vi "Begin.vi"(11 "Image Size":T1=enum."320x240") -> (0 "error out":errorcluster)   [LabVIEW 2012]
doc: "Called before other user functions, this VI is expected to open initial I/O refnums, load in file data, and do all program initialization. Notice that the <B>error out</B> terminal is simply used for data flow. Wiring it to other structures or subVIs ensures that this VI runs first."
uses:
  <vilib>/Rock Robotics/WPI/Camera/WPI_CameraImageSize.ctl
  <vilib>/Rock Robotics/WPI/DriverStation/WPI_DriverStationRobotMode2.ctl
  <vilib>/Rock Robotics/WPI/Joystick/WPI_JoystickDeviceEnum.ctl
  <vilib>/Rock Robotics/SystemInterfaces/DIO/FPGA_DIOPWMChannel.ctl
  <vilib>/Rock Robotics/SystemInterfaces/DIO/FPGA_DIORelayChannel.ctl
  <vilib>/Rock Robotics/SystemInterfaces/DIO/FPGA_DIOChannel.ctl
  <vilib>/Rock Robotics/SystemInterfaces/Typedef/FPGA_TypedefDigitalModule.ctl
  <vilib>/Rock Robotics/WPI/Encoder/WPI_EncoderType.ctl
  <vilib>/Rock Robotics/WPI/Solenoid/WPI_SolenoidChannel.ctl
  <vilib>/Rock Robotics/SystemInterfaces/Typedef/FPGA_TypedefAnalogModule.ctl
  <vilib>/Rock Robotics/SystemInterfaces/AI/FPGA_AIChannel.ctl
  RefnameEnum.ctl
  Sally_Dashboard_2014/DBNameEnum.ctl
  <vilib>/Rock Robotics/WPI/Solenoid/WPI_SolenoidValue.ctl
  <vilib>/Rock Robotics/WPI/SafetyOutput/WPI_SafetyOutputConfigMenu.ctl
  <vilib>/Rock Robotics/SystemInterfaces/CounterEncoderSourceConvertion/FPGA_CounterEncoderSourceConvertionLVSourceType.ctl
  <vilib>/Rock Robotics/SystemInterfaces/DIO/FPGA_DIODigitalSourceChannel.ctl
  <vilib>/Rock Robotics/SystemInterfaces/AnalogTrigger/FPGA_AnalogTriggerIndex.ctl
  <vilib>/Rock Robotics/SystemInterfaces/AnalogTrigger/FPGA_AnalogTriggerOutType.ctl
  Robot Global Data.vi
  <vilib>/Rock Robotics/WPI/RobotDrive/WPI_RobotDriveOpen2MotorWithTalon.vi
  <vilib>/Rock Robotics/WPI/MotorControl/WPI_MotorControlOpen Talon.vi
  <vilib>/Rock Robotics/WPI/Counter/WPI_CounterDigitalInputToDigitalSource.vi
  <vilib>/Rock Robotics/WPI/Solenoid/WPI_SolenoidOpenSingle.vi
  <vilib>/Rock Robotics/WPI/Solenoid/WPI_SolenoidSetEnum.vi
  <vilib>/Rock Robotics/WPI/MotorControl/WPI_MotorControlOpen Jaguar.vi
  <vilib>/Rock Robotics/WPI/Compressor/WPI_CompressorGetSetRefNum.vi
  <vilib>/Rock Robotics/WPI/Counter/WPI_CounterOpen UpDown Mode.vi
  <vilib>/Rock Robotics/WPI/Camera/WPI_CameraWhite Balance Values.ctl
  <vilib>/Rock Robotics/WPI/Camera/WPI_CameraExposure Values.ctl
  <vilib>/Rock Robotics/WPI/Camera/WPI_CameraFrameRate.ctl
  <vilib>/Rock Robotics/SystemInterfaces/Typedef/FPGA_TypedefAnalogModuleForGyro.ctl
  <vilib>/Rock Robotics/SystemInterfaces/AI/FPGA_AIGyroChannel.ctl
panel:
  in  "LowerLimit (v)":dbl=-1.0
  in  "UpperLimit (v)":dbl=1.0
  out "error out 2":errorcluster
  in  "Version String":string="TruongFramework 1.42"
  # "DON'T FORGET TO MAKE THIS DEFAULT"
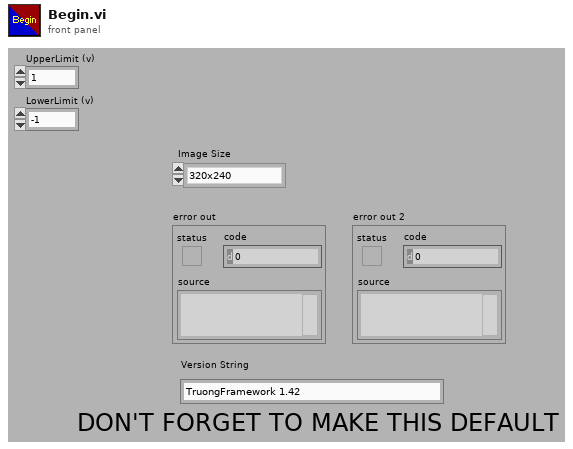
[diagram p1: front panel]
types:
  T1 = typedef "WPI_CameraImageSize.ctl" = enum16{"640x480", "320x240", "160x120"}
  T2 = typedef "WPI_SafetyOutputConfigMenu.ctl" = enum16{"Enable", "Disable"}
  T3 = typedef "WPI_SolenoidValue.ctl" = enum16{"Off", "On", "Forward", "Reverse"}
  T4 = typedef "RefnameEnum.ctl" = enum16{"FireLauncher", "Climber", "Shield", "TankDrive", "DriveEncoderL", "DriveEncoderR", "LauncherMotorRPM", "LauncherEncoderAnalog", "LauncherEncoderRPM", "ShooterLS", "DriveAlignLSLeft", "DriveAlignLSRight", "ClimbingLS", "LauncherEncoderAngle", "LauncherMotorAngle", "Gamepad1", "Gamepad2", "Compressor", "ClimbWeightSol3", "ClimbWeightSol4"}
  T5 = typedef "WPI_SolenoidChannel.ctl" = enum8{"Solenoid 1", "Solenoid 2", "Solenoid 3", "Solenoid 4", "Solenoid 5", "Solenoid 6", "Solenoid 7", "Solenoid 8", "Invalid"}
  T6 = typedef "FPGA_DIOChannel.ctl" = enum8{"DIO 1", "DIO 2", "DIO 3", "DIO 4", "DIO 5", "DIO 6", "DIO 7", "DIO 8", "DIO 9", "DIO 10", "DIO 11", "DIO 12", "DIO 13", "DIO 14", "Invalid"}
  T7 = typedef "FPGA_TypedefDigitalModule.ctl" = enum16{"Digital Module 1", "Digital Module 2"}
  T8 = typedef "DBNameEnum.ctl" = enum16{"AutoInstructions", "DriveLoopTime", "DriveAlignLSLeft", "DriveAlignLSRight", "Use2DriveAlign", "ClimbLS", "LauncherAngleMatches", "FrameworkVersion", "sLauncherAngle", "LauncherTargetAngle", "sLauncherRPM", "LauncherTargetRPM", "sDriveDistance", "LauncherMotorValue", "PullbackTol", "FireTol", "LauncherRPMTol", "LauncherAngleTol", "InitialWait", "WaitBetweenLaunch", "AnglePresets", "RPMPresets", "UseAngleEncoder", "UseLauncherEncoder", "UseLauncherPID", "QSWaitBeforeFire", "QSWaitBeforeRetract", "AngleForwardValue", "AngleBackwardValue", "UseClusterArray", "BackupAuto", "ReverseDriveIndicate", "HalfSpeedFactor"}
  T9 = typedef "FPGA_AIChannel.ctl" = enum8{"AI 1", "AI 2", "AI 3", "AI 4", "AI 5", "AI 6", "AI 7", "AI 8", "Invalid"}
  T10 = typedef "FPGA_TypedefAnalogModule.ctl" = enum16{"Analog Module 1", "Analog Module 2"}
  T11 = typedef "WPI_EncoderType.ctl" = enum16{"1x", "2x", "4x"}
  T12 = typedef "FPGA_DIORelayChannel.ctl" = enum8{"Relay 1", "Relay 2", "Relay 3", "Relay 4", "Relay 5", "Relay 6", "Relay 7", "Relay 8", "Invalid"}
  T13 = typedef "FPGA_DIOPWMChannel.ctl" = enum8{"PWM 1", "PWM 2", "PWM 3", "PWM 4", "PWM 5", "PWM 6", "PWM 7", "PWM 8", "PWM 9", "PWM 10", "Invalid"}
  T14 = typedef "WPI_JoystickDeviceEnum.ctl" = enum16{"USB 1", "USB 2", "USB 3", "USB 4", "Kinect 1", "Kinect 2"}
  T15 = typedef "WPI_DriverStationRobotMode2.ctl" = enum16{"Autonomous Disabled", "Autonomous Enabled", "Teleop Disabled", "Teleop Enabled", "Timeout", "Finish", "Test Disabled", "Test Enabled"}
  T16 = enum16{"Rising Edge", "Falling Edge", "Raising & Falling Edge", "Disabled"}
  T17 = typedef "WPI_DigitalInputDevRef.ctl" = cluster{"DevStatus":errorcluster, "DIO Channel":T6, "Digital Module":T7}
  T18 = typedef "FPGA_CounterEncoderSourceConvertionLVSourceType.ctl" = cluster{"DevStatus":errorcluster, "AnalogTriggerMode?":bool, "DigitalMode":cluster{"Digital Module":T7, "DIO Channel":T19}, "AnalogTriggerMode":cluster{"AnalogTriggerIndex":T20, "OutputType":T21}}
  T19 = typedef "FPGA_DIODigitalSourceChannel.ctl" = enum8{"DIO 1", "DIO 2", "DIO 3", "DIO 4", "DIO 5", "DIO 6", "DIO 7", "DIO 8", "DIO 9", "DIO 10", "DIO 11", "DIO 12", "DIO 13", "DIO 14", "Disabled"}
  T20 = typedef "FPGA_AnalogTriggerIndex.ctl" = enum8{"Trig 0", "Trig 1", "Trig 2", "Trig 3", "Trig 4", "Trig 5", "Trig 6", "Trig 7", "Invalid"}
  T21 = typedef "FPGA_AnalogTriggerOutType.ctl" = enum16{"InWindow", "TriggerState", "Rising", "Falling"}
  T22 = typedef "WPI_EncoderDevRef.ctl" = cluster{"DevStatus":errorcluster, "EncoderIndex":T23, "CounterIndex":T24, "DistancePerCount":dbl, "Decoding Type":T11}
  T23 = typedef "FPGA_EncoderIdx.ctl" = enum8{"Enc 0", "Enc 1", "Enc 2", "Enc 3", "Invalid"}
  T24 = typedef "FPGA_CounterCtrSystemIndex.ctl" = enum8{"Ctr 0", "Ctr 1", "Ctr 2", "Ctr 3", "Ctr 4", "Ctr 5", "Ctr 6", "Ctr 7", "Invalid"}
  T25 = typedef "WPI_CounterDevRef.ctl" = cluster{"DevStatus":errorcluster, "CntIndex":T24}
  T26 = typedef "FPGA_AIGyroChannel.ctl" = enum8{"AI 1", "AI 2", "Invalid"}
  T27 = typedef "FPGA_TypedefAnalogModuleForGyro.ctl" = enum16{"Analog Module 1"}
  T28 = typedef "WPI_GyroDevRef.ctl" = cluster{"DevStatus":errorcluster, "Analog Module":T10, "Analog Channel":T9, "Offset":dbl, "Gain (VoltsPerDegree/Second)":dbl}
  T29 = typedef "WPI_MotorControlDeviceRef.ctl" = cluster{"DeviceStatus":errorcluster, "Type":enum16{"PWM", "CAN"}, "PWM":cluster{"Digital Module":T7, "PWM Channel":T13, "DeadBand":T30}, "CAN":cluster{"Device Number":u8, "Control Mode":T31, "Semaphore":T32, "Max Vout":dbl}, "Invert":bool, "TransformRef":T33, "InvTransformRef":T33}
  T30 = typedef "WPI_PWMDeadband.ctl" = cluster{"Name":string, "maxPositivePwm":i32, "minPositivePwm":i32, "centerPwm":i32, "maxNegativePwm":i32, "minNegativePwm":i32, "angularRange":u16}
  T31 = typedef "WPI_CANJaguar_ControlMode.ctl" = enum8{"Percent VBus", "Current", "Speed", "Position", "Voltage"}
  T32 = typedef "Semaphore RefNum" = refnum<k1>
  T33 = typedef "WPI_PWMTransform_ConPane.ctl" = refnum<vi>
  T34 = typedef "WPI_RelayDevRef.ctl" = cluster{"DevStatus":errorcluster, "Relay Channel":T12, "Digital Module":T7, "Relay Direction":T35}
  T35 = typedef "WPI_RelayDirection.ctl" = enum16{"Both directions", "Forward only", "Reverse only"}
  T36 = typedef "WPI_SolenoidDevRef.ctl" = cluster{"DevStatus":errorcluster, "Solenoid Module":T37, "Forward Solenoid Channel":T5, "Reverse Solenoid Channel":T5}
  T37 = typedef "FPGA_TypedefSolenoidModule.ctl" = enum16{"Solenoid Module 1", "Solenoid Module 2"}
  T38 = typedef "WPI_CompressorDevRef.ctl" = cluster{"DevStatus":errorcluster, "DigitalInputDevRef":T17, "RelayDevRef":T34}
  T39 = typedef "WPI_RobotDriveDevRef.ctl" = cluster{"DevStatus":errorcluster, "Motors[]":T29[], "Square Inputs":bool, "Max Output":dbl, "Isochronous":bool}
  T40 = typedef "WPI_CameraFrameRate.ctl" = u32
  T41 = typedef "WPI_CameraExposure Values.ctl" = enum16{"Auto", "Flicker-free 50 Hz", "Flicker-free 60 Hz", "Hold current"}
  T42 = typedef "WPI_CameraWhite Balance Values.ctl" = enum16{"Auto", "Fixed indoor", "Fixed outdoor 1", "Fixed outdoor 2", "Fixed fluorescent 1", "Fixed fluorescent 2", "Hold current"}
  T43 = typedef "WPI_CameraDevRef.ctl" = cluster{"Camera Address":string, "CameraStatus":errorcluster, "Acquire Image Notifier":refnum<notifier>}
  T44 = typedef "WPI_JoystickDevRef.ctl" = cluster{"Device":T14}
  T45 = typedef "WPI_AnalogChannelDevRef.ctl" = cluster{"DevStatus":errorcluster, "Analog Module":T10, "Analog Channel":T9}
  T46 = typedef "FPGA_AnalogTriggerDevRef.ctl" = cluster{"DevStatus":errorcluster, "AnalogTriggerIndex":T20}
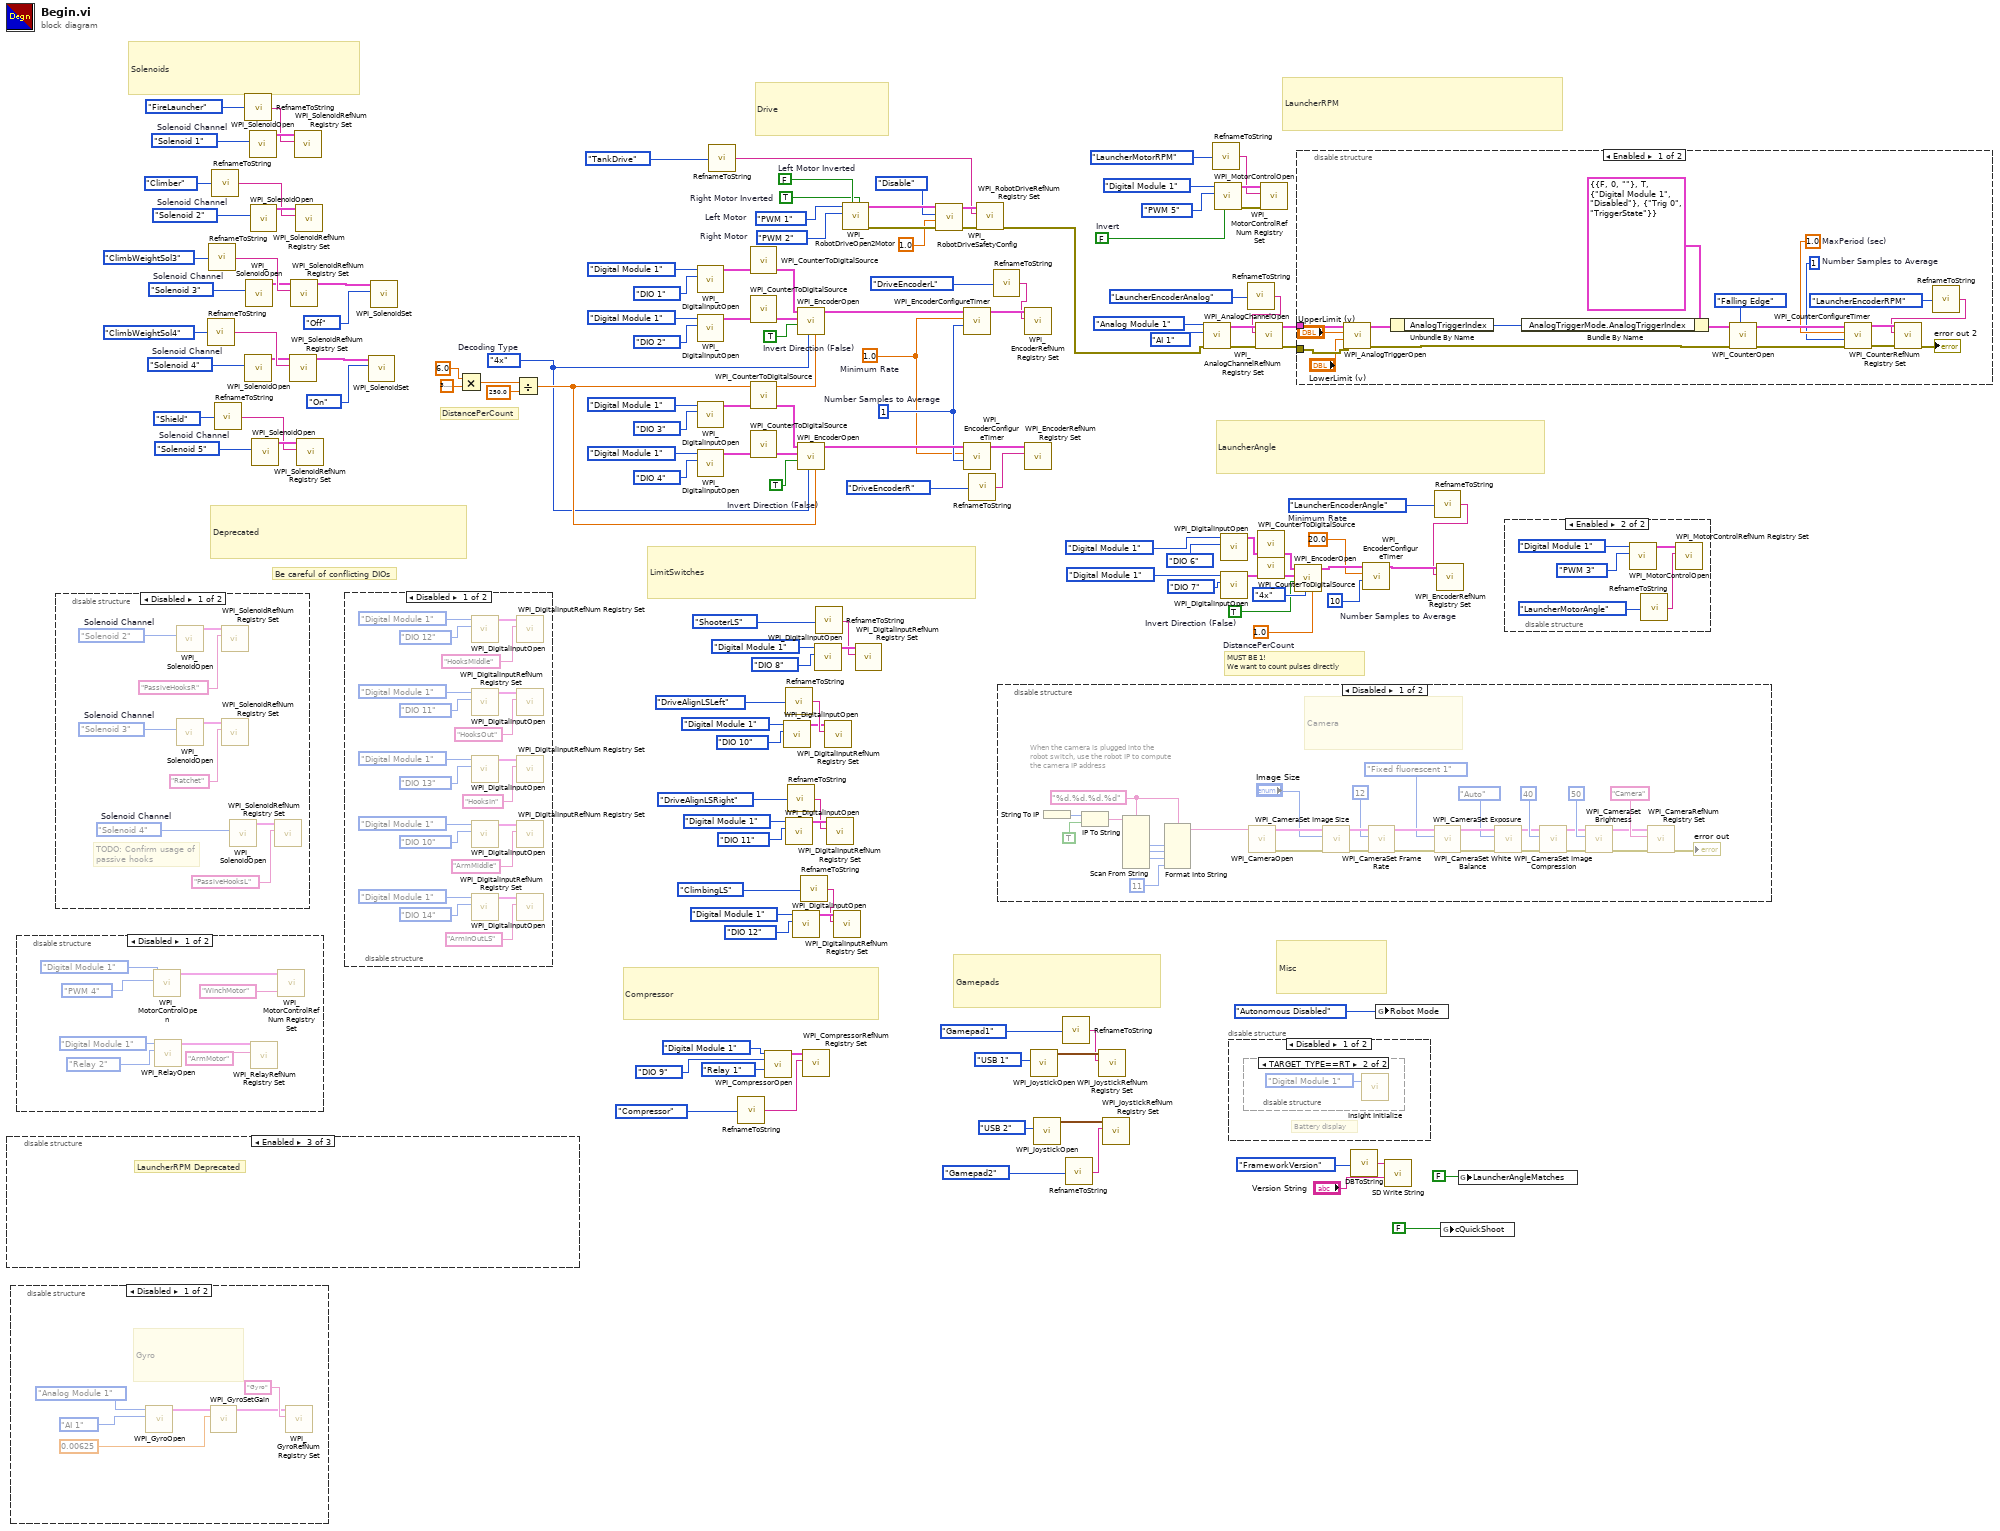
[diagram p0: block diagram]
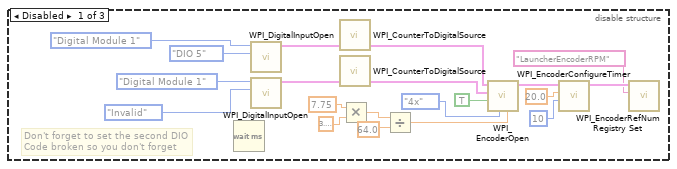
[diagram p8: hidden frame]
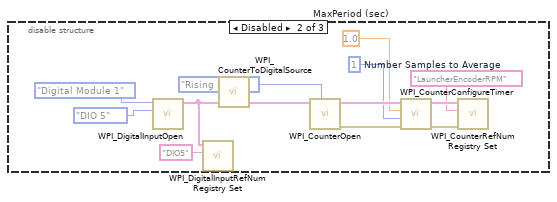
[diagram p9: hidden frame]
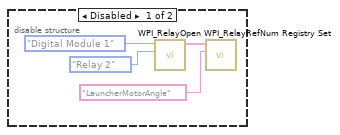
[diagram p12: hidden frame]
diagram:
  w12 = WPI_SolenoidChannel."Solenoid 4"  # Solenoid Channel
  w16 = WPI_SolenoidChannel."Solenoid 3"  # Solenoid Channel
  w72 = 1.0  # DistancePerCount
  w75 = TRUE  # Invert Direction (False)
  w76 = TRUE  # Invert Direction (False)
  w80 = WPI_SolenoidChannel."Solenoid 5"  # Solenoid Channel
  w82 = WPI_SolenoidChannel."Solenoid 2"  # Solenoid Channel
  w87 = TRUE  # Invert Direction (False)
  w89 = u8 10  # Number Samples to Average
  w90 = 20.0  # Minimum Rate
  w102 = WPI_SolenoidChannel."Solenoid 1"  # Solenoid Channel
  w77 = WPI_EncoderType."4x"  # Decoding Type
  w74 = u8 1  # Number Samples to Average
  w73 = 1.0  # Minimum Rate
  w131 = FALSE  # Invert
  w135 = FPGA_DIOPWMChannel."PWM 2"  # Right Motor
  w136 = FPGA_DIOPWMChannel."PWM 1"  # Left Motor
  w137 = TRUE  # Right Motor Inverted
  w138 = FALSE  # Left Motor Inverted
  # "Be careful of conflicting DIOs"
  # "DistancePerCount"
  # "Deprecated"
  # "LimitSwitches"
  # "Compressor"
  # "Solenoids"
  # "LauncherAngle"
  # "LauncherRPM"
  # "Misc"
  # "Gamepads"
  # "Drive"
  # "MUST BE 1!\nWe want to count pulses directly"
  n1 = disable-structure shown="Enabled" {
    frame Disabled {
      # "Don't forget to set the second DIO\nCode broken so you don't forget"
      n2 = Wait (ms)() -> ()  [unwired: 1 in, 1 out]
      n3 = call <vilib>:"WPI_DigitalInputOpen.vi"("DIO Channel"=FPGA_DIOChannel."DIO 5", "Digital Module (Module 1)"=FPGA_TypedefDigitalModule."Digital Module 1") -> ("DigitalInputDevRef"=w161:T17)  [unwired: 1 in, 8 out]
      n4 = call <vilib>:"WPI_DigitalInputOpen.vi"("DIO Channel"=FPGA_DIOChannel."Invalid", "Digital Module (Module 1)"=FPGA_TypedefDigitalModule."Digital Module 1") -> ("DigitalInputDevRef"=w162:T17)  [unwired: 1 in, 8 out]
      n5 = call-poly <vilib>:"WPI_CounterToDigitalSource.vi"("DigitalInputDevRef"=w161) -> ("Digital Source"=w160:T18)  [unwired: 6 out]
      n6 = call-poly <vilib>:"WPI_CounterToDigitalSource.vi"("DigitalInputDevRef"=w162) -> ("Digital Source"=w163:T18)  [unwired: 6 out]
      n7 = Multiply(x=7.75, y=3.141592653589793) -> (x*y=w145:dbl)
      n8 = Divide(x=w145, y=64.0) -> (x/y=w148:dbl)
      n9 = call <vilib>:"WPI_EncoderOpen.vi"("DistancePerCount"=w148, "Decoding Type"=WPI_EncoderType."4x", "Invert Direction (False)"=TRUE, "BSource"=w163, "ASource"=w160) -> ("EncoderDevRef"=w157:T22)  [unwired: 3 in, 3 out]
      n10 = call <vilib>:"WPI_EncoderConfigureTimer.vi"("Number Samples to Average"=u8 10, "Minimum Rate"=20.0, "EncoderDevRef"=w157) -> ("EncoderDevRef"=w154:T22)  [unwired: 1 in, 7 out]
      n11 = call <vilib>:"WPI_EncoderRefNum Registry Set.vi"("refnum name"="LauncherEncoderRPM", "EncoderDevRef"=w154) -> ()  [unwired: 8 in, 2 out]
    }
    frame Disabled {
      w174 = u8 1  # Number Samples to Average
      w175 = 1.0  # MaxPeriod (sec)
      n12 = call <vilib>:"WPI_DigitalInputOpen.vi"("DIO Channel"=FPGA_DIOChannel."DIO 5", "Digital Module (Module 1)"=FPGA_TypedefDigitalModule."Digital Module 1") -> ("DigitalInputDevRef"=w165:T17)  [unwired: 8 in, 1 out]
      n13 = call <vilib>:"WPI_DigitalInputRefNum Registry Set.vi"("refnum name"="DIO5", "DigitalInputDevRef"=w165) -> ()  [unwired: 8 in, 2 out]
      n14 = call-poly <vilib>:"WPI_CounterToDigitalSource.vi"("DigitalInputDevRef"=w165) -> ("Digital Source"=w168:T18)  [unwired: 6 out]
      n15 = call-poly <vilib>:"WPI_CounterOpen.vi"("UpEdge"=T16."Rising Edge", "Up Source"=w168) -> ("error out"=w170:errorcluster, "CounterDevRef"=w176:T25)  [unwired: 8 in]
      n16 = call <vilib>:"WPI_CounterConfigureTimer.vi"("error in (no error)"=w170, "Number Samples to Average"=w174, "MaxPeriod (sec)"=w175, "CounterDevRef in"=w176) -> ("error out"=w169:errorcluster, "CounterDevRef out"=w173:T25)  [unwired: 6 in]
      n17 = call <vilib>:"WPI_CounterRefNum Registry Set.vi"("error in (no error)"=w169, "refnum name"="LauncherEncoderRPM", "CounterDevRef"=w173) -> ()  [unwired: 7 in, 2 out]
    }
    frame Enabled {
      # "LauncherRPM Deprecated"
    }
  }
  n18 = disable-structure shown="Disabled" {
    frame Disabled {
      # "Gyro"
      n19 = call <vilib>:"WPI_GyroOpen.vi"("Analog Channel"=FPGA_AIGyroChannel."AI 1", "Analog Module (Module 1)"=FPGA_TypedefAnalogModuleForGyro."Analog Module 1") -> ("GyroDevRef"=w179:T28)  [unwired: 7 in, 2 out]
      n20 = call <vilib>:"WPI_GyroSetGain.vi"("Gain (VoltsPerDegree/Second)"=0.00625, "GyroDevRef"=w179) -> ("GyroDevRef"=w178:T28)  [unwired: 8 in, 1 out]
      n21 = call <vilib>:"WPI_GyroRefNum Registry Set.vi"("refnum name"="Gyro", "GyroDevRef"=w178) -> ()  [unwired: 8 in, 2 out]
    }
    frame Enabled {
    }
  }
  n22 = disable-structure shown="Disabled" {
    frame Disabled {
      n23 = call-poly <vilib>:"WPI_MotorControlOpen.vi"("PWM Channel"=FPGA_DIOPWMChannel."PWM 4", "Digital Module (Module 1)"=FPGA_TypedefDigitalModule."Digital Module 1") -> ("MotorControlDeviceRef"=w188:T29)  [unwired: 8 in, 1 out]
      n24 = call <vilib>:"WPI_RelayOpen.vi"("Relay Channel"=FPGA_DIORelayChannel."Relay 2", "Digital Module (Module 1)"=FPGA_TypedefDigitalModule."Digital Module 1") -> ("RelayDevRef"=w184:T34)  [unwired: 8 in, 1 out]
      n25 = call <vilib>:"WPI_RelayRefNum Registry Set.vi"("refnum name"="ArmMotor", "RelayDevRef"=w184) -> ()  [unwired: 8 in, 2 out]
      n26 = call <vilib>:"WPI_MotorControlRefNum Registry Set.vi"("refnum name"="WinchMotor", "MotorControlDevRef"=w188) -> ()  [unwired: 8 in, 2 out]
    }
    frame Enabled {
    }
  }
  n27 = disable-structure shown="Disabled" {
    frame Disabled {
      w193 = WPI_SolenoidChannel."Solenoid 2"  # Solenoid Channel
      w196 = WPI_SolenoidChannel."Solenoid 4"  # Solenoid Channel
      w199 = WPI_SolenoidChannel."Solenoid 3"  # Solenoid Channel
      # "TODO: Confirm usage of\npassive hooks"
      n28 = call-poly <vilib>:"WPI_SolenoidOpen.vi"("Solenoid Channel"=w193) -> ("SolenoidDevRef"=w192:T36)  [unwired: 2 in, 8 out]
      n29 = call-poly <vilib>:"WPI_SolenoidOpen.vi"("Solenoid Channel"=w199) -> ("SolenoidDevRef"=w198:T36)  [unwired: 2 in, 8 out]
      n30 = call <vilib>:"WPI_SolenoidRefNum Registry Set.vi"("refnum name"="PassiveHooksR", "SolenoidDevRef"=w192) -> ()  [unwired: 8 in, 2 out]
      n31 = call <vilib>:"WPI_SolenoidRefNum Registry Set.vi"("refnum name"="Ratchet", "SolenoidDevRef"=w198) -> ()  [unwired: 8 in, 2 out]
      n32 = call-poly <vilib>:"WPI_SolenoidOpen.vi"("Solenoid Channel"=w196) -> ("SolenoidDevRef"=w195:T36)  [unwired: 2 in, 8 out]
      n33 = call <vilib>:"WPI_SolenoidRefNum Registry Set.vi"("refnum name"="PassiveHooksL", "SolenoidDevRef"=w195) -> ()  [unwired: 8 in, 2 out]
    }
    frame Enabled {
    }
  }
  n34 = call "RefnameToString.vi"("Enum"=RefnameEnum."ClimbWeightSol4") -> ("Refname"=w15:string)
  n35 = call "RefnameToString.vi"("Enum"=RefnameEnum."ClimbWeightSol3") -> ("Refname"=w19:string)
  n36 = call "RefnameToString.vi"("Enum"=RefnameEnum."Climber") -> ("Refname"=w53:string)
  n37 = call "RefnameToString.vi"("Enum"=RefnameEnum."Shield") -> ("Refname"=w51:string)
  n38 = call "RefnameToString.vi"("Enum"=RefnameEnum."FireLauncher") -> ("Refname"=w55:string)
  n39 = call-poly <vilib>:"WPI_SolenoidOpen.vi"("Solenoid Channel"=w12) -> ("SolenoidDevRef"=w13:T36)  [unwired: 2 in, 8 out]
  n40 = call-poly <vilib>:"WPI_SolenoidOpen.vi"("Solenoid Channel"=w16) -> ("SolenoidDevRef"=w17:T36)  [unwired: 2 in, 8 out]
  n41 = call-poly <vilib>:"WPI_SolenoidOpen.vi"("Solenoid Channel"=w102) -> ("SolenoidDevRef"=w101:T36)  [unwired: 2 in, 8 out]
  n42 = call-poly <vilib>:"WPI_SolenoidOpen.vi"("Solenoid Channel"=w82) -> ("SolenoidDevRef"=w81:T36)  [unwired: 2 in, 8 out]
  n43 = call-poly <vilib>:"WPI_SolenoidOpen.vi"("Solenoid Channel"=w80) -> ("SolenoidDevRef"=w79:T36)  [unwired: 2 in, 8 out]
  n44 = call <vilib>:"WPI_SolenoidRefNum Registry Set.vi"("refnum name"=w15, "SolenoidDevRef"=w13) -> ("SolenoidDevRef"=w10:T36)  [unwired: 8 in, 1 out]
  n45 = call <vilib>:"WPI_SolenoidRefNum Registry Set.vi"("refnum name"=w19, "SolenoidDevRef"=w17) -> ("SolenoidDevRef"=w11:T36)  [unwired: 8 in, 1 out]
  n46 = call <vilib>:"WPI_SolenoidRefNum Registry Set.vi"("refnum name"=w55, "SolenoidDevRef"=w101) -> ()  [unwired: 8 in, 2 out]
  n47 = call <vilib>:"WPI_SolenoidRefNum Registry Set.vi"("refnum name"=w53, "SolenoidDevRef"=w81) -> ()  [unwired: 8 in, 2 out]
  n48 = call <vilib>:"WPI_SolenoidRefNum Registry Set.vi"("refnum name"=w51, "SolenoidDevRef"=w79) -> ()  [unwired: 8 in, 2 out]
  n49 = disable-structure shown="Disabled" {
    frame Disabled {
      n50 = call <vilib>:"WPI_DigitalInputOpen.vi"("DIO Channel"=FPGA_DIOChannel."DIO 12", "Digital Module (Module 1)"=FPGA_TypedefDigitalModule."Digital Module 1") -> ("DigitalInputDevRef"=w203:T17)  [unwired: 8 in, 1 out]
      n51 = call <vilib>:"WPI_DigitalInputOpen.vi"("DIO Channel"=FPGA_DIOChannel."DIO 11", "Digital Module (Module 1)"=FPGA_TypedefDigitalModule."Digital Module 1") -> ("DigitalInputDevRef"=w207:T17)  [unwired: 8 in, 1 out]
      n52 = call <vilib>:"WPI_DigitalInputOpen.vi"("DIO Channel"=FPGA_DIOChannel."DIO 13", "Digital Module (Module 1)"=FPGA_TypedefDigitalModule."Digital Module 1") -> ("DigitalInputDevRef"=w211:T17)  [unwired: 8 in, 1 out]
      n53 = call <vilib>:"WPI_DigitalInputOpen.vi"("DIO Channel"=FPGA_DIOChannel."DIO 10", "Digital Module (Module 1)"=FPGA_TypedefDigitalModule."Digital Module 1") -> ("DigitalInputDevRef"=w215:T17)  [unwired: 8 in, 1 out]
      n54 = call <vilib>:"WPI_DigitalInputOpen.vi"("DIO Channel"=FPGA_DIOChannel."DIO 14", "Digital Module (Module 1)"=FPGA_TypedefDigitalModule."Digital Module 1") -> ("DigitalInputDevRef"=w219:T17)  [unwired: 8 in, 1 out]
      n55 = call <vilib>:"WPI_DigitalInputRefNum Registry Set.vi"("refnum name"="HooksMiddle", "DigitalInputDevRef"=w203) -> ()  [unwired: 8 in, 2 out]
      n56 = call <vilib>:"WPI_DigitalInputRefNum Registry Set.vi"("refnum name"="HooksOut", "DigitalInputDevRef"=w207) -> ()  [unwired: 8 in, 2 out]
      n57 = call <vilib>:"WPI_DigitalInputRefNum Registry Set.vi"("refnum name"="HooksIn", "DigitalInputDevRef"=w211) -> ()  [unwired: 8 in, 2 out]
      n58 = call <vilib>:"WPI_DigitalInputRefNum Registry Set.vi"("refnum name"="ArmMiddle", "DigitalInputDevRef"=w215) -> ()  [unwired: 8 in, 2 out]
      n59 = call <vilib>:"WPI_DigitalInputRefNum Registry Set.vi"("refnum name"="ArmInOutLS", "DigitalInputDevRef"=w219) -> ()  [unwired: 8 in, 2 out]
    }
    frame Enabled {
    }
  }
  n60 = call-poly <vilib>:"WPI_SolenoidSet.vi"("Value"=WPI_SolenoidValue."On", "SolenoidDevRef"=w10) -> ()  [unwired: 8 in, 2 out]
  n61 = call-poly <vilib>:"WPI_SolenoidSet.vi"("Value"=WPI_SolenoidValue."Off", "SolenoidDevRef"=w11) -> ()  [unwired: 8 in, 2 out]
  n62 = Multiply(x=6.0, y=3.141592653589793) -> (x*y=w84:dbl)
  n63 = Divide(x=w84, y=250.0) -> (x/y=w78:dbl)
  n64 = call <vilib>:"WPI_DigitalInputOpen.vi"("DIO Channel"=FPGA_DIOChannel."DIO 1", "Digital Module (Module 1)"=FPGA_TypedefDigitalModule."Digital Module 1") -> ("DigitalInputDevRef"=w123:T17)  [unwired: 1 in, 8 out]
  n65 = call <vilib>:"WPI_DigitalInputOpen.vi"("DIO Channel"=FPGA_DIOChannel."DIO 2", "Digital Module (Module 1)"=FPGA_TypedefDigitalModule."Digital Module 1") -> ("DigitalInputDevRef"=w124:T17)  [unwired: 1 in, 8 out]
  n66 = call <vilib>:"WPI_DigitalInputOpen.vi"("DIO Channel"=FPGA_DIOChannel."DIO 3", "Digital Module (Module 1)"=FPGA_TypedefDigitalModule."Digital Module 1") -> ("DigitalInputDevRef"=w110:T17)  [unwired: 1 in, 8 out]
  n67 = call <vilib>:"WPI_DigitalInputOpen.vi"("DIO Channel"=FPGA_DIOChannel."DIO 4", "Digital Module (Module 1)"=FPGA_TypedefDigitalModule."Digital Module 1") -> ("DigitalInputDevRef"=w111:T17)  [unwired: 1 in, 8 out]
  n68 = call "RefnameToString.vi"("Enum"=RefnameEnum."TankDrive") -> ("Refname"=w3:string)
  n69 = call "RefnameToString.vi"("Enum"=RefnameEnum."Compressor") -> ("Refname"=w32:string)
  n70 = call-poly <vilib>:"WPI_CounterToDigitalSource.vi"("DigitalInputDevRef"=w123) -> ("Digital Source"=w122:T18)  [unwired: 6 out]
  n71 = call-poly <vilib>:"WPI_CounterToDigitalSource.vi"("DigitalInputDevRef"=w124) -> ("Digital Source"=w125:T18)  [unwired: 6 out]
  n72 = call-poly <vilib>:"WPI_CounterToDigitalSource.vi"("DigitalInputDevRef"=w110) -> ("Digital Source"=w109:T18)  [unwired: 6 out]
  n73 = call-poly <vilib>:"WPI_CounterToDigitalSource.vi"("DigitalInputDevRef"=w111) -> ("Digital Source"=w112:T18)  [unwired: 6 out]
  n74 = call <vilib>:"WPI_CompressorOpen.vi"("Pressure Switch Digital Module (Module 1)"=FPGA_TypedefDigitalModule."Digital Module 1" ("Pressure Switch\nand Relay Module"), "Pressure Switch DIO Channel"=FPGA_DIOChannel."DIO 9" ("Pressure Switch Channel"), "Relay Channel"=FPGA_DIORelayChannel."Relay 1") -> ("CompressorDevRef"=w126:T38)  [unwired: 2 in, 10 out]
  n75 = call <vilib>:"WPI_DigitalInputOpen.vi"("DIO Channel"=FPGA_DIOChannel."DIO 10", "Digital Module (Module 1)"=FPGA_TypedefDigitalModule."Digital Module 1") -> ("DigitalInputDevRef"=w21:T17)  [unwired: 8 in, 1 out]
  n76 = call "RefnameToString.vi"("Enum"=RefnameEnum."DriveAlignLSLeft") -> ("Refname"=w25:string)
  n77 = call <vilib>:"WPI_DigitalInputOpen.vi"("DIO Channel"=FPGA_DIOChannel."DIO 11", "Digital Module (Module 1)"=FPGA_TypedefDigitalModule."Digital Module 1") -> ("DigitalInputDevRef"=w65:T17)  [unwired: 8 in, 1 out]
  n78 = call "RefnameToString.vi"("Enum"=RefnameEnum."DriveAlignLSRight") -> ("Refname"=w36:string)
  n79 = call <vilib>:"WPI_DigitalInputOpen.vi"("DIO Channel"=FPGA_DIOChannel."DIO 12", "Digital Module (Module 1)"=FPGA_TypedefDigitalModule."Digital Module 1") -> ("DigitalInputDevRef"=w59:T17)  [unwired: 8 in, 1 out]
  n80 = call <vilib>:"WPI_EncoderOpen.vi"("DistancePerCount"=w78, "Decoding Type"=w77, "Invert Direction (False)"=w76, "BSource"=w125, "ASource"=w122) -> ("EncoderDevRef"=w119:T22)  [unwired: 3 in, 3 out]
  n81 = call <vilib>:"WPI_EncoderOpen.vi"("DistancePerCount"=w78, "Decoding Type"=w77, "Invert Direction (False)"=w75, "BSource"=w112, "ASource"=w109) -> ("EncoderDevRef"=w106:T22)  [unwired: 3 in, 3 out]
  n82 = call "RefnameToString.vi"("Enum"=RefnameEnum."ClimbingLS") -> ("Refname"=w34:string)
  n83 = call <vilib>:"WPI_CompressorRefNum Registry Set.vi"("refnum name"=w32, "CompressorDevRef"=w126) -> ()  [unwired: 8 in, 2 out]
  n84 = call <vilib>:"WPI_DigitalInputOpen.vi"("DIO Channel"=FPGA_DIOChannel."DIO 8", "Digital Module (Module 1)"=FPGA_TypedefDigitalModule."Digital Module 1") -> ("DigitalInputDevRef"=w115:T17)  [unwired: 8 in, 1 out]
  n85 = call "RefnameToString.vi"("Enum"=RefnameEnum."ShooterLS") -> ("Refname"=w38:string)
  n86 = call <vilib>:"WPI_DigitalInputRefNum Registry Set.vi"("refnum name"=w25, "DigitalInputDevRef"=w21) -> ()  [unwired: 8 in, 2 out]
  n87 = call <vilib>:"WPI_DigitalInputRefNum Registry Set.vi"("refnum name"=w36, "DigitalInputDevRef"=w65) -> ()  [unwired: 8 in, 2 out]
  n88 = call <vilib>:"WPI_DigitalInputRefNum Registry Set.vi"("refnum name"=w34, "DigitalInputDevRef"=w59) -> ()  [unwired: 8 in, 2 out]
  n89 = call-poly <vilib>:"WPI_RobotDriveOpen2Motor.vi"("Right Motor Inverted"=w137, "Left Motor Inverted"=w138, "Right Motor"=w135, "Left Motor"=w136) -> ("error out"=w4:errorcluster, "RobotDriveDevRef"=w7:T39)  [unwired: 6 in]
  n90 = call <vilib>:"WPI_DigitalInputRefNum Registry Set.vi"("refnum name"=w38, "DigitalInputDevRef"=w115) -> ()  [unwired: 8 in, 2 out]
  n91 = call <vilib>:"WPI_RobotDriveSafetyConfig.vi"("error in (no error)"=w4, "timeout (s)"=1.0, "mode"=WPI_SafetyOutputConfigMenu."Disable", "RobotDriveDevRef"=w7) -> ("error out"=w5:errorcluster, "RobotDriveDevRef"=w6:T39)  [unwired: 6 in]
  n92 = call <vilib>:"WPI_EncoderConfigureTimer.vi"("Number Samples to Average"=w74, "Minimum Rate"=w73, "EncoderDevRef"=w119) -> ("EncoderDevRef"=w116:T22)  [unwired: 1 in, 7 out]
  n93 = call <vilib>:"WPI_EncoderConfigureTimer.vi"("Number Samples to Average"=w74, "Minimum Rate"=w73, "EncoderDevRef"=w106) -> ("EncoderDevRef"=w103:T22)  [unwired: 1 in, 7 out]
  n94 = call "RefnameToString.vi"("Enum"=RefnameEnum."DriveEncoderR") -> ("Refname"=w46:string)
  n95 = call <vilib>:"WPI_RobotDriveRefNum Registry Set.vi"("error in (no error)"=w5, "refnum name"=w3, "RobotDriveDevRef"=w6) -> ("error out"=w62:errorcluster)  [unwired: 7 in, 1 out]
  n96 = call "RefnameToString.vi"("Enum"=RefnameEnum."DriveEncoderL") -> ("Refname"=w48:string)
  n97 = disable-structure shown="Disabled" {
    frame Disabled {
      w222 = "%d.%d.%d.%d" ("format string")
      # "Camera"
      # "When the camera is plugged into the\nrobot switch, use the robot IP to compute\nthe camera IP address"
      n98 = String To IP() -> (0:w229:u32)  [unwired: 1 in]
      n99 = IP To String(1:TRUE ("dot notation? (F)"), 2:w229) -> (0:w227:string)
      n100 = Scan From String(format string=w222, input string=w227) -> (output 1=w226:i32, output 2=w225:i32, output 3=w224:i32)  [unwired: 7 in, 3 out]
      n101 = Format Into String(format string=w222, w226, w225, w224, 11 ("Compression")) -> (resulting string=w221:string)  [unwired: 2 in, 1 out]
      n102 = call <vilib>:"WPI_CameraOpen.vi"("Camera Address"=w221) -> ("error out"=w241:errorcluster, "CameraDevRef"=w242:T43)  [unwired: 1 in, 8 out]
      n103 = call <vilib>:"WPI_CameraSet Image Size.vi"("error in (no error)"=w241, "Image Size"="Image Size", "CameraDevRef"=w242) -> ("error out"=w240:errorcluster, "CameraDevRef Out"=w243:T43)  [unwired: 7 out]
      n104 = call <vilib>:"WPI_CameraSet Frame Rate.vi"("error in (no error)"=w240, "Frame Rate (fps)"=T40 12, "CameraDevRef"=w243) -> ("error out"=w239:errorcluster, "CameraDevRef Out"=w245:T43)  [unwired: 7 out]
      n105 = call <vilib>:"WPI_CameraSet White Balance.vi"("error in (no error)"=w239, "White Balance"=WPI_CameraWhite_Balance_Values."Fixed fluorescent 1", "CameraDevRef"=w245) -> ("error out"=w238:errorcluster, "CameraDevRef Out"=w244:T43)  [unwired: 7 out]
      n106 = call <vilib>:"WPI_CameraSet Exposure.vi"("error in (no error)"=w238, "Exposure"=WPI_CameraExposure_Values."Auto", "CameraDevRef"=w244) -> ("error out"=w237:errorcluster, "CameraDevRef Out"=w247:T43)  [unwired: 7 out]
      n107 = call <vilib>:"WPI_CameraSet Image Compression.vi"("error in (no error)"=w237, "Compression"=40, "CameraDevRef"=w247) -> ("error out"=w236:errorcluster, "CameraDevRef Out"=w246:T43)  [unwired: 7 out]
      n108 = call <vilib>:"WPI_CameraSet Brightness.vi"("error in (no error)"=w236, "Brightness"=50, "CameraDevRef"=w246) -> ("error out"=w234:errorcluster, "CameraDevRef Out"=w235:T43)  [unwired: 7 out]
      n109 = call <vilib>:"WPI_CameraRefNum Registry Set.vi"("error in (no error)"=w234, "refnum name"="Camera", "CameraDevRef"=w235) -> ("error out"=→"error out":errorcluster)  [unwired: 8 out]
    }
    frame Enabled {
    }
  }
  n110 = call <vilib>:"WPI_EncoderRefNum Registry Set.vi"("refnum name"=w48, "EncoderDevRef"=w116) -> ()  [unwired: 8 in, 2 out]
  n111 = call <vilib>:"WPI_EncoderRefNum Registry Set.vi"("refnum name"=w46, "EncoderDevRef"=w103) -> ()  [unwired: 8 in, 2 out]
  n112 = call <vilib>:"WPI_JoystickOpen.vi"("JoystickDevice"=WPI_JoystickDeviceEnum."USB 1") -> ("JoystickDevRef"=w142:T44)  [unwired: 10 in]
  n113 = call <vilib>:"WPI_JoystickOpen.vi"("JoystickDevice"=WPI_JoystickDeviceEnum."USB 2") -> ("JoystickDevRef"=w139:T44)  [unwired: 10 in]
  n114 = call "RefnameToString.vi"("Enum"=RefnameEnum."Gamepad1") -> ("Refname"=w28:string)
  n115 = call "RefnameToString.vi"("Enum"=RefnameEnum."Gamepad2") -> ("Refname"=w30:string)
  n116 = call <vilib>:"WPI_JoystickRefNum Registry Set.vi"("refnum name"=w28, "JoystickDevRef"=w142) -> ()  [unwired: 8 in, 2 out]
  n117 = call <vilib>:"WPI_JoystickRefNum Registry Set.vi"("refnum name"=w30, "JoystickDevRef"=w139) -> ()  [unwired: 8 in, 2 out]
  n118 = call <vilib>:"WPI_AnalogChannelOpen.vi"("error in (no error)"=w62, "Analog Channel"=FPGA_AIChannel."AI 1", "Analog Module (Module 1)"=FPGA_TypedefAnalogModule."Analog Module 1") -> ("error out"=w67:errorcluster, "AIDeviceRef"=w66:T45)  [unwired: 7 in]
  n119 = call "RefnameToString.vi"("Enum"=RefnameEnum."LauncherMotorRPM") -> ("Refname"=w44:string)
  n120 = call-poly <vilib>:"WPI_MotorControlOpen.vi"("Invert"=w131, "PWM Channel"=FPGA_DIOPWMChannel."PWM 5", "Digital Module (Module 1)"=FPGA_TypedefDigitalModule."Digital Module 1") -> ("error out"=w130:errorcluster, "MotorControlDeviceRef"=w134:T29)  [unwired: 7 in]
  n121 = call <vilib>:"WPI_DigitalInputOpen.vi"("DIO Channel"=FPGA_DIOChannel."DIO 6", "Digital Module (Module 1)"=FPGA_TypedefDigitalModule."Digital Module 1") -> ("DigitalInputDevRef"=w98:T17)  [unwired: 1 in, 8 out]
  n122 = call <vilib>:"WPI_DigitalInputOpen.vi"("DIO Channel"=FPGA_DIOChannel."DIO 7", "Digital Module (Module 1)"=FPGA_TypedefDigitalModule."Digital Module 1") -> ("DigitalInputDevRef"=w99:T17)  [unwired: 1 in, 8 out]
  n123 = disable-structure shown="Disabled" {
    frame Disabled {
      # "Battery display"
      n124 = disable-structure shown="TARGET_TYPE==RT" {
        frame condition #0 {
        }
        frame condition #1 (active) {
          n125 = call "Insight Initialize.vi"("Digital Module"=FPGA_TypedefDigitalModule."Digital Module 1") -> ()  [unwired: 2 in]
        }
      }
    }
    frame Enabled {
    }
  }
  n126 = call "RefnameToString.vi"("Enum"=RefnameEnum."LauncherEncoderAnalog") -> ("Refname"=w42:string)
  n127 = call <vilib>:"WPI_AnalogChannelRefNum Registry Set.vi"("error in (no error)"=w67, "refnum name"=w42, "AIDeviceRef"=w66) -> ("error out"=w60:errorcluster, "AIDeviceRef"=w61:T45)  [unwired: 7 in]
  n128 = call-poly <vilib>:"WPI_CounterToDigitalSource.vi"("DigitalInputDevRef"=w98) -> ("Digital Source"=w97:T18)  [unwired: 6 out]
  n129 = call-poly <vilib>:"WPI_CounterToDigitalSource.vi"("DigitalInputDevRef"=w99) -> ("Digital Source"=w100:T18)  [unwired: 6 out]
  n130 = call <vilib>:"WPI_MotorControlRefNum Registry Set.vi"("error in (no error)"=w130, "refnum name"=w44, "MotorControlDevRef"=w134) -> ()  [unwired: 7 in, 2 out]
  n131 = call <vilib>:"WPI_EncoderOpen.vi"("DistancePerCount"=w72, "Decoding Type"=WPI_EncoderType."4x", "Invert Direction (False)"=w87, "BSource"=w100, "ASource"=w97) -> ("EncoderDevRef"=w94:T22)  [unwired: 3 in, 3 out]
  n132 = disable-structure shown="Enabled" {
    disable-tunnel: w61 -> [w257 _]
    disable-tunnel: w60 -> [w256 _]
    frame Enabled {
      w266 = u8 1  # Number Samples to Average
      w267 = 1.0  # MaxPeriod (sec)
      n133 = call <vilib>:"WPI_AnalogTriggerOpen.vi"("error in (no error)"=w256, "LowerLimit (v)"="LowerLimit (v)", "UpperLimit (v)"="UpperLimit (v)", "AnalogTriggerSource"=w257) -> ("error out"=w270:errorcluster, "AnalogTriggerDevRef"=w265:T46)  [unwired: 6 in]
      n134 = Unbundle By Name(w265) -> ("AnalogTriggerIndex"=w264:T20)
      n135 = Bundle By Name(cluster=T18 {"DevStatus"={"status"=FALSE, "code"=0, "source"=""}, "AnalogTriggerMode?"=TRUE, "DigitalMode"={"Digital Module"=enum."Digital Module 1", "DIO Channel"=enum."Disabled"}, "AnalogTriggerMode"={"AnalogTriggerIndex"=enum."Trig 0", "OutputType"=enum."TriggerState"}} ("Source"), "AnalogTriggerMode.AnalogTriggerIndex"=w264) -> (w262:T18)
      n136 = call-poly <vilib>:"WPI_CounterOpen.vi"("UpEdge"=T16."Falling Edge" ("UpEdge 1"), "error in (no error)"=w270, "Up Source"=w262) -> ("error out"=w268:errorcluster, "CounterDevRef"=w269:T25)  [unwired: 7 in]
      n137 = call <vilib>:"WPI_CounterConfigureTimer.vi"("error in (no error)"=w268, "Number Samples to Average"=w266, "MaxPeriod (sec)"=w267, "CounterDevRef in"=w269) -> ("error out"=w259:errorcluster, "CounterDevRef out"=w260:T25)  [unwired: 6 in]
      n138 = call "RefnameToString.vi"("Enum"=RefnameEnum."LauncherEncoderRPM") -> ("Refname"=w254:string)
      n139 = call <vilib>:"WPI_CounterRefNum Registry Set.vi"("error in (no error)"=w259, "refnum name"=w254, "CounterDevRef"=w260) -> ("error out"=→"error out 2":errorcluster)  [unwired: 7 in, 1 out]
    }
    frame Disabled {
    }
  }
  n140 = call "DBToString.vi"("Enum"=DBNameEnum."FrameworkVersion") -> ("Refname"=w26:string)
  n141 = call <vilib>:"WPI_EncoderConfigureTimer.vi"("Number Samples to Average"=w89, "Minimum Rate"=w90, "EncoderDevRef"=w94) -> ("EncoderDevRef"=w91:T22)  [unwired: 1 in, 7 out]
  n142 = global write "Robot Global Data.vi" "Robot Mode"(WPI_DriverStationRobotMode2."Autonomous Disabled" ("Robot Mode")) -> ()
  n143 = call <vilib>:"SD Write String.vi"("String"="Version String", "Name"=w26) -> ()  [unwired: 8 in, 2 out]
  n144 = call "RefnameToString.vi"("Enum"=RefnameEnum."LauncherEncoderAngle") -> ("Refname"=w40:string)
  n145 = call <vilib>:"WPI_EncoderRefNum Registry Set.vi"("refnum name"=w40, "EncoderDevRef"=w91) -> ()  [unwired: 8 in, 2 out]
  n146 = global write "Robot Global Data.vi" "cQuickShoot"(FALSE) -> ()
  n147 = global write "Robot Global Data.vi" "LauncherAngleMatches"(FALSE) -> ()
  n148 = disable-structure shown="Enabled" {
    frame Disabled {
      n149 = call <vilib>:"WPI_RelayOpen.vi"("Relay Channel"=FPGA_DIORelayChannel."Relay 2", "Digital Module (Module 1)"=FPGA_TypedefDigitalModule."Digital Module 1") -> ("RelayDevRef"=w272:T34)  [unwired: 8 in, 1 out]
      n150 = call <vilib>:"WPI_RelayRefNum Registry Set.vi"("refnum name"="LauncherMotorAngle", "RelayDevRef"=w272) -> ()  [unwired: 8 in, 2 out]
    }
    frame Enabled {
      n151 = call-poly <vilib>:"WPI_MotorControlOpen.vi"("PWM Channel"=FPGA_DIOPWMChannel."PWM 3", "Digital Module (Module 1)"=FPGA_TypedefDigitalModule."Digital Module 1") -> ("MotorControlDeviceRef"=w278:T29)  [unwired: 8 in, 1 out]
      n152 = call "RefnameToString.vi"("Enum"=RefnameEnum."LauncherMotorAngle") -> ("Refname"=w275:string)
      n153 = call <vilib>:"WPI_MotorControlRefNum Registry Set.vi"("refnum name"=w275, "MotorControlDevRef"=w278) -> ()  [unwired: 8 in, 2 out]
    }
  }
